vi "myPython.vi"() -> ()   [LabVIEW 2019]
uses:
  3bc521ba-1157-4ca2-8ff3-c98ad85f0d40.vi
  8f3016a3-c5d1-4f0b-92cf-39b4cc4eb427.vi
  <vilib>/Utility/sysdir.llb/Get System Directory.vi
panel:
  in  "Tab Control":T1(tab)
  in  "a":dbl=41.0
  in  "b":dbl=1.0
  out "a + b":dbl
  in  "a 3":dbl=41.0
  in  "b 3":dbl=1.0
  out "a + b 2":dbl
  in  "b":i32=1
  in  "a":i32=41
  out "a + b":i32
  in  "array":i32[](array[numeric])=[1, 2, 3]
  in  "new element":i32=4
  out "modified array":i32[](array[numeric])
  in  "str1":string="Hello "
  in  "str2":string="World"
  out "concatenated string":string
  in  "a 2":dbl[][](array[numeric])=[[1.0, 2.0, 3.0], [4.0, 5.0, 6.0], [7.0, 8.0, 9.0]]
  in  "b 2":dbl[][](array[numeric])=[[1.0, 0.0, 0.0], [0.0, 1.0, 0.0], [0.0, 0.0, 1.0]]
  out "a*b":dbl[][](array[numeric])
  out "<JSON>":string
  out "result":i32[](array[numeric])
  in  "Numeric":i32=100 format="%.0p"
  out "create JSON":dbl format="%#_6p"
  out "parse JSON":dbl format="%#_6p"
  out "open Python session":dbl format="%#_6p"
  out "total":dbl
  out "error out":errorcluster
  in  "error in (no error)":errorcluster
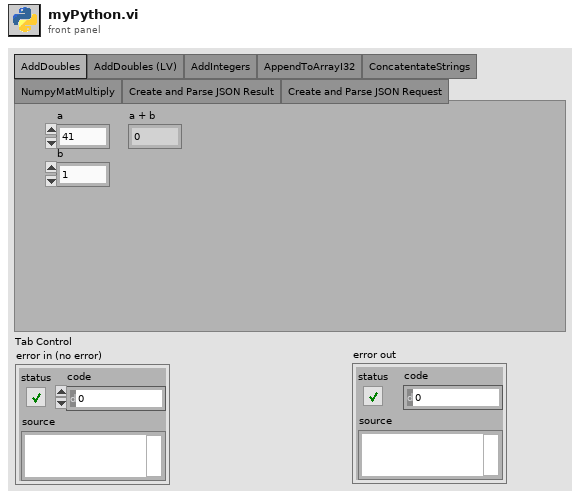
[diagram p1: front panel]
types:
  T1 = enum32{"AddDoubles", "AddDoubles (LV)", "AddIntegers", "AppendToArrayI32", "ConcatentateStrings", "NumpyMatMultiply", "Create and Parse JSON Result", "Create and Parse JSON Request"}
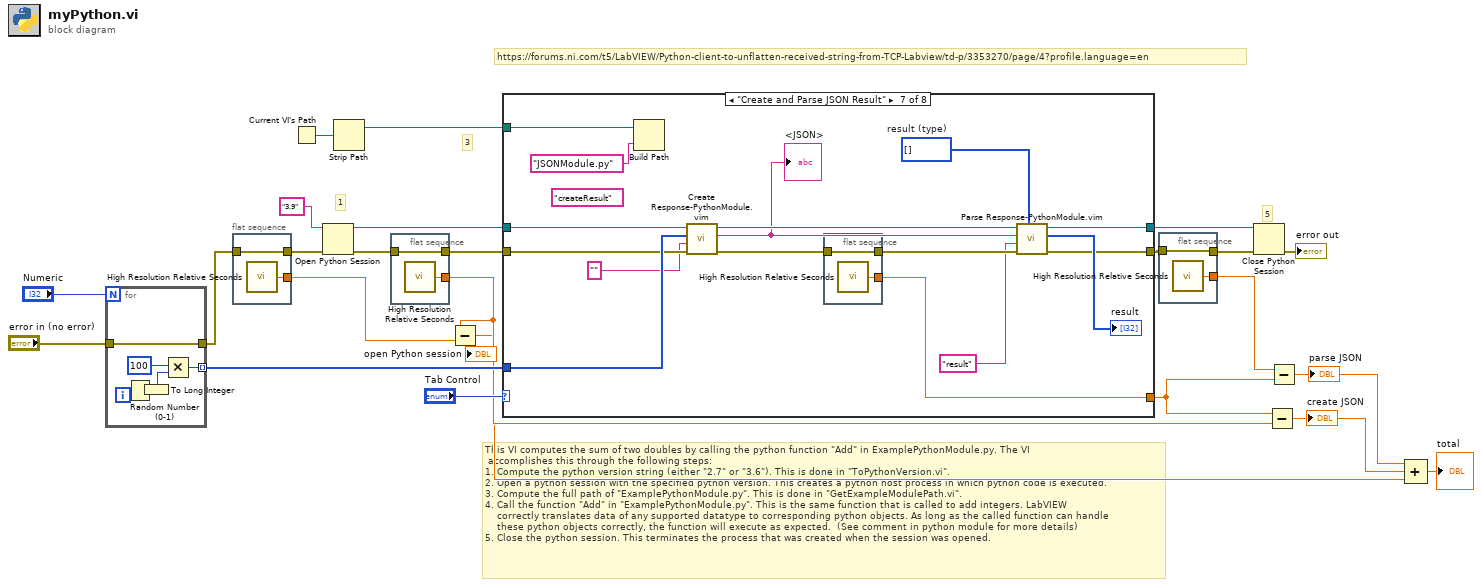
[diagram p0: block diagram]
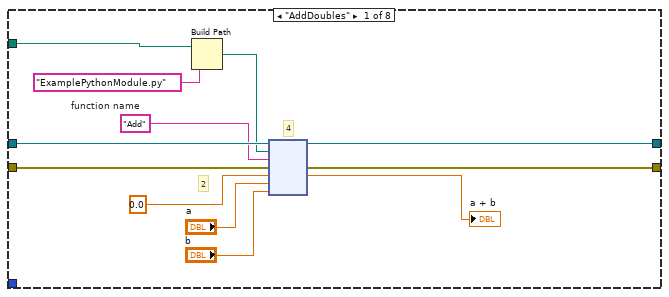
[diagram p2: hidden frame]
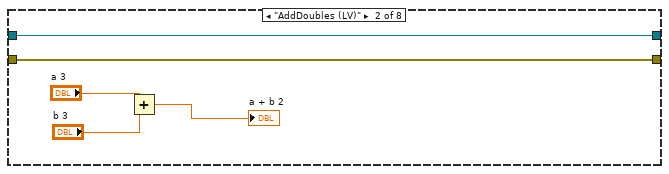
[diagram p3: hidden frame]
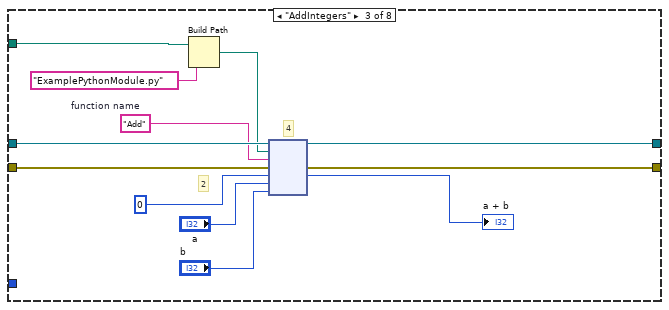
[diagram p4: hidden frame]
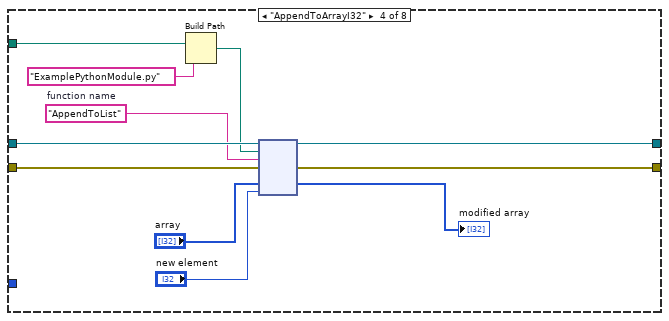
[diagram p5: hidden frame]
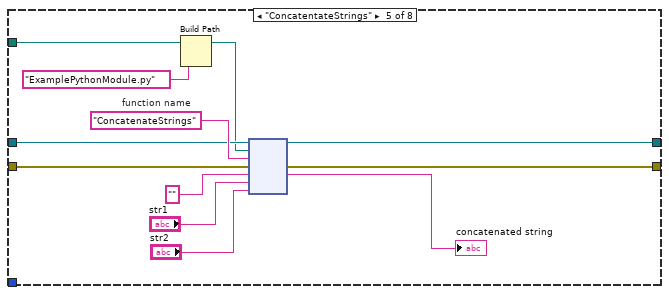
[diagram p6: hidden frame]
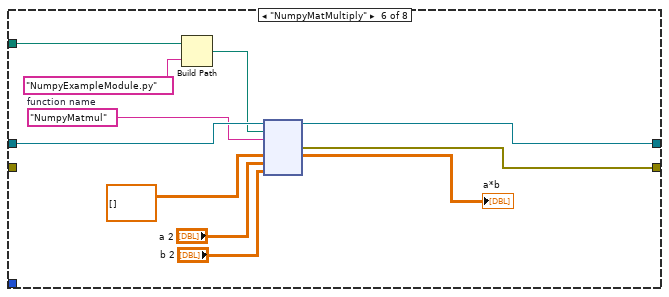
[diagram p7: hidden frame]
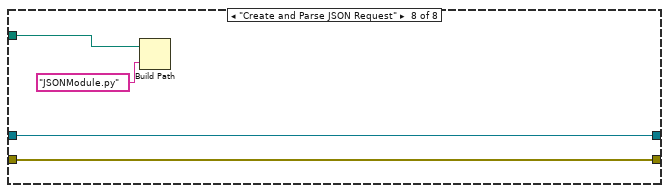
[diagram p8: hidden frame]
diagram:
  # "https://forums.ni.com/t5/LabVIEW/Python-client-to-unflatten-received-string-from-TCP-Labview/td-p/3353270/page/4?profile.language=en"
  # "5"
  # "3"
  # "1"
  # "This VI computes the sum of two doubles by calling the python function \"Add\" in ExamplePythonModule.py. The VI\n accomplishes this through the following steps:\n1. Compute the python version string (either \"2.7\" or \"3.6\"). This is done in \"ToPythonVersion.vi\". \n2. Open a python session with the specified python version. This creates a python host process in which python code is executed.\n3. Compute the full path of \"ExamplePythonModule.py\". This is done in \"GetExampleModulePath.vi\".\n4. Call the function \"Add\" in \"ExamplePythonModule.py\". This is the same function that is called to add integers. LabVIEW \n    correctly translates data of any supported datatype to corresponding python objects. As long as the called function can handle\n    these python objects correctly, the function will execute as expected.  (See comment in python module for more details)\n5. Close the python session. This terminates the process that was created when the session was opened."
  n1 = for {
    N: "Numeric" -> [_]
    tunnel: [w28] -> w14 mode=indexing
    tunnel: "error in (no error)" -> [w26]
    tunnel: [w26] -> w7
    n2 = Random Number (0-1)() -> (number: 0 to 1=w27:dbl)
    n3 = To Long Integer(number=w27) -> (32bit integer=w25:i32)
    n4 = Multiply(x=100, y=w25) -> (x*y=w28:i32)
  }
  n5 = flat-sequence {
    tunnel: [w31] -> w9
    tunnel: w7 -> [w31]
    tunnel: [w30] -> w8
    frame #0 {
      n6 = call <vilib>:"High Resolution Relative Seconds.vi"() -> ("relative seconds"=w30:dbl)
    }
  }
  n7 = Current VI's Path() -> (path=w23:path)
  n8 = Open Python Session(python version="3.9" ("Python version"), 3:w9) -> (session out=w17:refnum<k35>, error out=w19:errorcluster)  [unwired: 1 in]
  n9 = Strip Path(path=w23) -> (stripped path=w21:path)  [unwired: 1 out]
  n10 = flat-sequence {
    tunnel: [w33] -> w20
    tunnel: w19 -> [w33]
    tunnel: [w32] -> w10
    frame #0 {
      n11 = call <vilib>:"High Resolution Relative Seconds.vi"() -> ("relative seconds"=w32:dbl)
    }
  }
  n12 = Subtract(x=w10, y=w8) -> (x-y=w3:dbl)
  "open Python session" <- w3
  n13 = case shown="\"Create and Parse JSON Result\"" "Tab Control" {
    tunnel: w17 -> [w45 w49 w62 w73 w81 w94 w108 w114]
    tunnel: w20 -> [w44 w50 w61 w72 w80 _ w106 w115]
    tunnel: [w42 w49 w59 w66 w78 w93 w102 w114] -> w15
    tunnel: [w41 w50 w58 w67 w79 w92 w96 w115] -> w16
    tunnel: w21 -> [w35 _ w52 w64 w76 w86 w110 w116]
    tunnel: w14 -> [_ _ _ _ _ _ w107 _]
    tunnel: [_ _ _ _ _ _ w109 _] -> w11
    frame "AddDoubles" {
      w43 = "Add"  # function name
      # "4"
      # "2"
      n14 = Build Path(base path=w35, name or relative path="ExamplePythonModule.py") -> (appended path=w34:path)
      n15 = node(w45, w34, w43, w44, 0.0 ("a"), "a", "b") -> (w42:refnum<k35>, w41:errorcluster, →"a + b":dbl)  [unwired: 2 in, 2 out]
    }
    frame "AddDoubles (LV)" {
      n16 = Add(x="a 3", y="b 3") -> (x+y=→"a + b 2":dbl)
    }
    frame "AddIntegers" {
      w60 = "Add"  # function name
      # "4"
      # "2"
      n17 = Build Path(base path=w52, name or relative path="ExamplePythonModule.py") -> (appended path=w51:path)
      n18 = node(w62, w51, w60, w61, 0 ("a"), "a", "b") -> (w59:refnum<k35>, w58:errorcluster, →"a + b":i32)  [unwired: 2 in, 2 out]
    }
    frame "AppendToArrayI32" {
      w71 = "AppendToList"  # function name
      n19 = Build Path(base path=w64, name or relative path="ExamplePythonModule.py") -> (appended path=w63:path)
      n20 = node(w73, w63, w71, w72, "array", "new element") -> (w66:refnum<k35>, w67:errorcluster, →"modified array":i32[])  [unwired: 3 in, 2 out]
    }
    frame "ConcatentateStrings" {
      w84 = "ConcatenateStrings"  # function name
      n21 = Build Path(name or relative path="ExamplePythonModule.py") -> ()  [unwired: 1 in, 1 out]
      n22 = node(w81, w76, w84, w80, "" ("str1"), "str1", "str2") -> (w78:refnum<k35>, w79:errorcluster, →"concatenated string":string)  [unwired: 2 in, 2 out]
    }
    frame "NumpyMatMultiply" {
      w88 = "NumpyMatmul"  # function name
      n23 = Build Path(base path=w86, name or relative path="NumpyExampleModule.py") -> (appended path=w85:path)
      n24 = node(w94, w85, w88, dbl[][] [] ("b"), "a 2", "b 2") -> (w93:refnum<k35>, w92:errorcluster, →"a*b":dbl[][])  [unwired: 3 in, 2 out]
    }
    frame "Create and Parse JSON Result" {
      w101 = i32[] []  # result (type)
      (unwired) "createResult" ("name or relative path")
      n25 = Build Path(base path=w110, name or relative path="JSONModule.py") -> ()  [unwired: 1 out]
      n26 = call "Create Response-PythonModule.vim"("error in (no error)"=w106, "id"="", "Response"=w107, "session in"=w108) -> ("error out"=w105:errorcluster, "{JSON}"=w100:string, "session out"=w103:refnum<k35>)  [unwired: 5 in]
      "<JSON>" <- w100
      n27 = flat-sequence {
        tunnel: [w113] -> w99
        tunnel: w105 -> [w113]
        tunnel: [w112] -> w109
        frame #0 {
          n28 = call <vilib>:"High Resolution Relative Seconds.vi"() -> ("relative seconds"=w112:dbl)
        }
      }
      n29 = call "Parse Response-PythonModule.vim"("Response Type"=w101, "error in (no error)"=w99, "Key"="result", "{JSON}"=w100, "session in"=w103) -> ("error out"=w96:errorcluster, "Response"=→"result":i32[], "session out"=w102:refnum<k35>)  [unwired: 4 in]
    }
    frame "Create and Parse JSON Request" {
      n30 = Build Path(base path=w116, name or relative path="JSONModule.py") -> ()  [unwired: 1 out]
    }
  }
  n31 = flat-sequence {
    tunnel: [w119] -> w18
    tunnel: w16 -> [w119]
    tunnel: [w118] -> w12
    frame #0 {
      n32 = call <vilib>:"High Resolution Relative Seconds.vi"() -> ("relative seconds"=w118:dbl)
    }
  }
  n33 = Close Python Session(session in=w15, error in=w18) -> (11:→"error out":errorcluster)
  n34 = Subtract(x=w11, y=w10) -> (x-y=w1:dbl)
  "create JSON" <- w1
  n35 = Subtract(x=w12, y=w11) -> (x-y=w4:dbl)
  "parse JSON" <- w4
  n36 = Compound Arithmetic op=ADD(w4, w1, w3) -> (→"total":dbl)
